vi "Populate Tree Items.vi"() -> ()   [LabVIEW 2023]
doc: "Demonstrates populating the items of the Tree control."
panel:
  in  "Third item attributes":string[](array[string])=["Sample 5", "Sample 6"]
  in  "Item indent level":i32[](array[numeric])=[0, 0, 1, 0, 0]
  in  "Second item attributes":string[](array[string])=["Sample 3", "Sample 4"]
  in  "Requested item tags":string[](array[string])=["One Tag", "Duplicate Tag", "Duplicate Tag"]
  in  "First item attributes":string[](array[string])=["Sample 1", "Sample 2"]
  out "Actual item tags (no duplicates)":string[](array[string])
  in  "Item names":string[](array[string])=["First item", "Duplicate", "Duplicate"]
  in  "Tree":string(tree)
  # "Overview: Demonstrates populating the items of the Tree control.\nInstructions:\n1. Run the VI to populate the Tree control.\n2. Open the block diagram for more information."
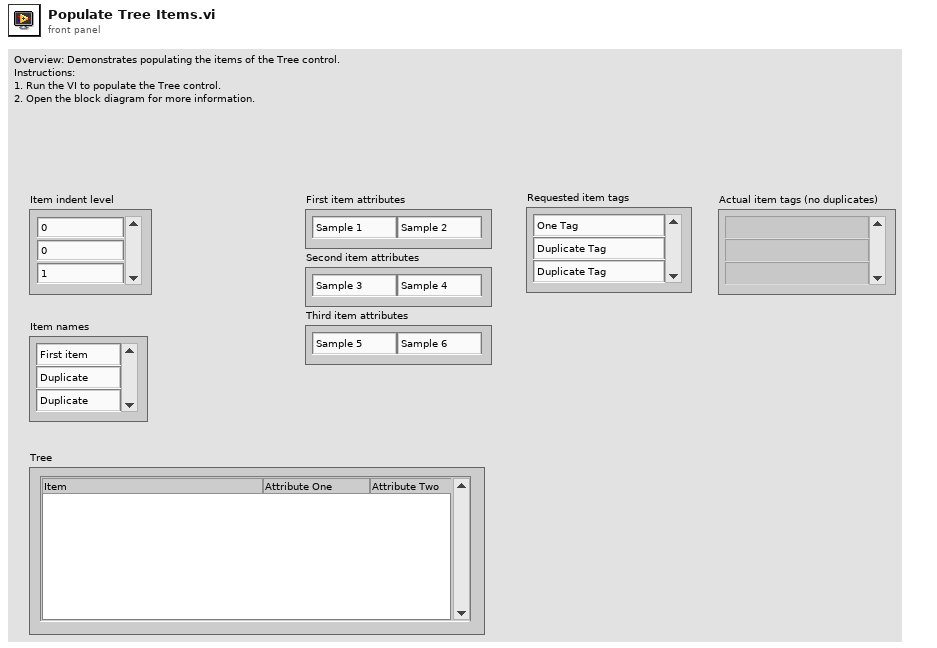
[diagram p1: front panel]
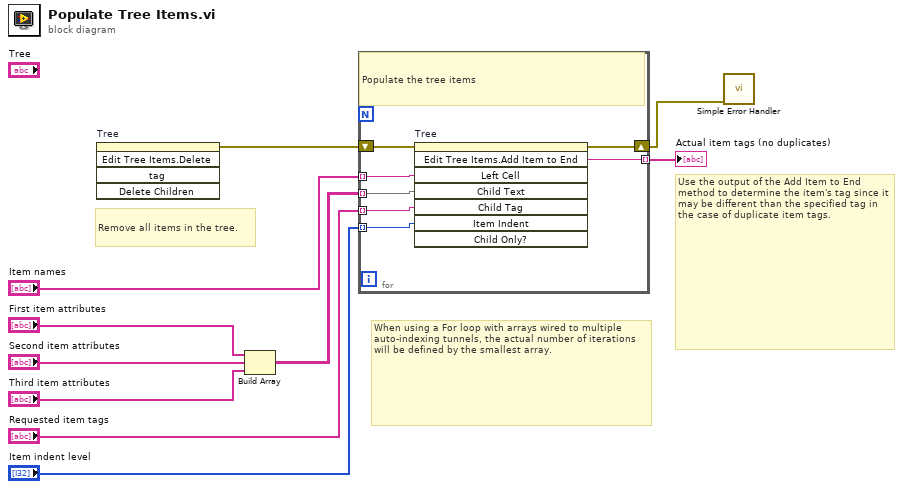
[diagram p0: block diagram]
diagram:
  # "When using a For loop with arrays wired to multiple auto-indexing tunnels, the actual number of iterations will be defined by the smallest array."
  # "Use the output of the Add Item to End method to determine the item's tag since it may be different than the specified tag in the case of duplicate item tags."
  # "Remove all items in the tree."
  n1 = invoke on="Tree" class="Tree (strict)" method="Edit Tree Items.Delete"() -> (error out=w10:errorcluster)  [unwired: 5 in, 4 out]
  n2 = Build Array("First item attributes", "Second item attributes", "Third item attributes") -> (w2:string[][])
  n3 = for {
    tunnel: "Item names" -> [w16] mode=indexing
    tunnel: [w15] -> w9 mode=indexing
    tunnel: "Requested item tags" -> [w14] mode=indexing
    tunnel: "Item indent level" -> [w13] mode=indexing
    tunnel: w2 -> [w11] mode=indexing
    shift-right: [w12] -> w3
    shift-left: w10 -> [w17]
    # "Populate the tree items"
    n4 = invoke on="Tree" class="Tree (strict)" method="Edit Tree Items.Add Item to End"(error in=w17, "Left Cell"=w16, "Child Text"=w11, "Child Tag"=w14, "Item Indent"=w13) -> (error out=w12:errorcluster, "Edit Tree Items:Add Item to End"=w15:string)  [unwired: 3 in, 6 out]
  }
  "Actual item tags (no duplicates)" <- w9
  n5 = call <vilib>:"Simple Error Handler.vi"("error in (no error)"=w3) -> ()  [unwired: 4 in, 5 out]
